vi "ex_CalcNewX0.vi"(7 "reset":bool, 8 "samples":i32[](array[numeric]), 10 "Delta X":dbl[](array[numeric]) format="%.2f", 11 "Initial X0":timestamp[](array[timestamp])) -> (3 "X0":timestamp[](array[timestamp]))   [LabVIEW 2020]
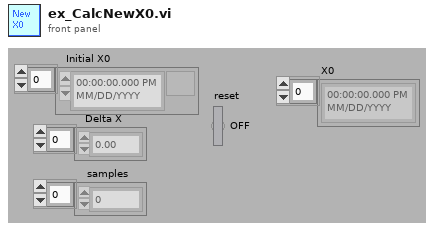
[diagram p1: front panel]
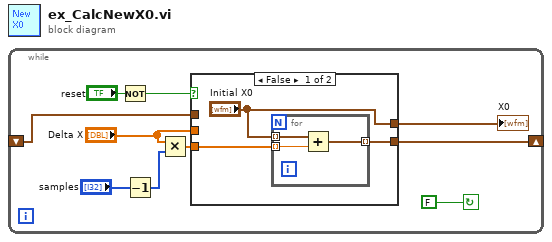
[diagram p0: block diagram]
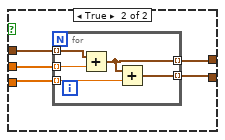
[diagram p2: hidden frame]
diagram:
  n1 = while {
    shift-right: [w4] -> _
    shift-left: _ -> [w3]
    stop <- FALSE continue-if-true
    n2 = Not(x="reset") -> (.not. x?=w1:bool)
    n3 = Decrement(x="samples") -> (x-1=w10:i32[])
    n4 = Multiply(x="Delta X", y=w10) -> (x*y=w9:dbl[])
    n5 = case shown="False" w1 {
      tunnel: w3 -> [_ w21]
      tunnel: ["Initial X0" w17] -> w8
      tunnel: "Delta X" -> [_ w20]
      tunnel: w9 -> [w13 w19]
      tunnel: [w12 w18] -> w4
      frame False {
        n6 = for {
          tunnel: w13 -> [w16] mode=indexing
          tunnel: [w15] -> w12 mode=indexing
          tunnel: "Initial X0" -> [w14] mode=indexing
          n7 = Add(x=w14, y=w16) -> (x+y=w15:timestamp)
        }
      }
      frame True {
        n8 = for {
          tunnel: w21 -> [w26] mode=indexing
          tunnel: w20 -> [w25] mode=indexing
          tunnel: w19 -> [w24] mode=indexing
          tunnel: [w23] -> w18 mode=indexing
          tunnel: [w22] -> w17 mode=indexing
          n9 = Add(x=w26, y=w25) -> (x+y=w22:timestamp)
          n10 = Add(x=w22, y=w24) -> (x+y=w23:timestamp)
        }
      }
    }
    "X0" <- w8
  }
